vi "Error Channels Read Array.vi"(8 "error in":errorcluster, 11 "Cycler in":refnum<class "Cycler.lvclass">) -> (0 "error out":errorcluster, 1 "Changed or First Call?":bool, 2 "Error Acknowledge Channels ACT":bool[](array[boolean]), 3 "Cycler out":refnum<class "Cycler.lvclass">)   [LabVIEW 2023, in "Cycler.lvclass"]
uses:
  Cycler.lvclass
  Cycler.lvclass/Cycler.ctl
  Low Level Capabilities/Error Channels/Error Channels.lvclass
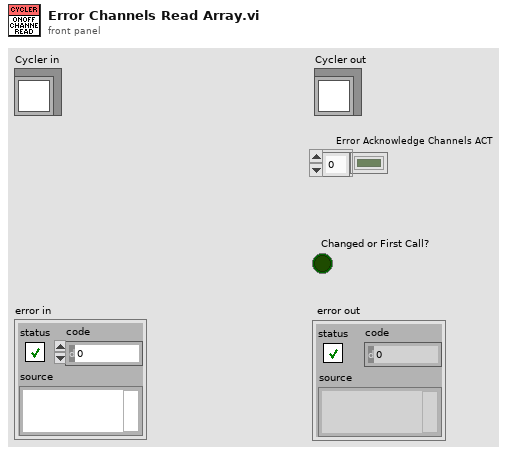
[diagram p1: front panel]
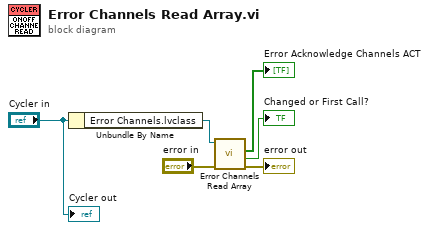
[diagram p0: block diagram]
diagram:
  n1 = Unbundle By Name("Cycler in") -> ("Error Channels.lvclass"=w1:refnum<class "Error Channels.lvclass">)
  n2 = call "Error Channels Read Array.vi"("error in"="error in", "Error Channels In"=w1) -> ("error out"=→"error out":errorcluster, "Changed or First Call?"=→"Changed or First Call?":bool, "Error Acknowledge Channels ACT"=→"Error Acknowledge Channels ACT":bool[])  [unwired: 6 in, 1 out]
  "Cycler out" <- "Cycler in"
